vi "loopTime.vi"(8 "error in (no error)":errorcluster, 11 "Model in":refnum<class "Model.lvclass">) -> (0 "error out":errorcluster, 2 "loop Time":dbl, 3 "Model out":refnum<class "Model.lvclass">)   [LabVIEW 2016, in "Model.lvclass"]
uses:
  Model.lvclass
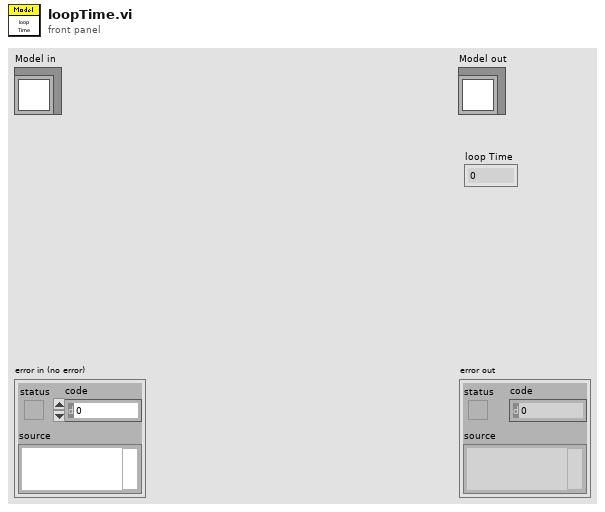
[diagram p1: front panel]
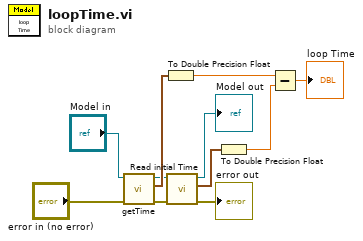
[diagram p0: block diagram]
diagram:
  n1 = call-dynamic "getTime.vi"("error in (no error)"="error in (no error)", "Model in"="Model in") -> ("error out"=w9:errorcluster, "Time Stamp"=w5:timestamp, "Model out"=w4:refnum<class "Model.lvclass">)  [unwired: 7 in]
  n2 = To Double Precision Float(number=w5) -> (double precision float=w6:dbl)
  n3 = call-dynamic "Read initial Time.vi"("error in (no error)"=w9, "Model in"=w4) -> ("error out"=→"error out":errorcluster, "initial Time"=w8:timestamp, "Model out"=→"Model out":refnum<class "Model.lvclass">)  [unwired: 7 in]
  n4 = To Double Precision Float(number=w8) -> (double precision float=w7:dbl)
  n5 = Subtract(x=w6, y=w7) -> (x-y=→"loop Time":dbl)
